vi "StopCore.vi"(8 "error in (no error)":errorcluster caption="错误输入（无错误）", 11 "zsActor输入":refnum<class "ActorWrapper.lvclass">) -> (0 "error out":errorcluster caption="错误输出", 3 "zsActor输出":refnum<class "ActorWrapper.lvclass">)   [LabVIEW 2014]
uses:
  zsActor/ActorWrapper.lvclass
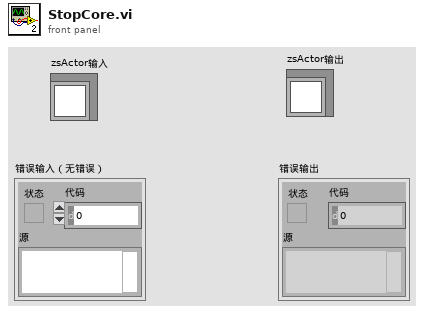
[diagram p1: front panel]
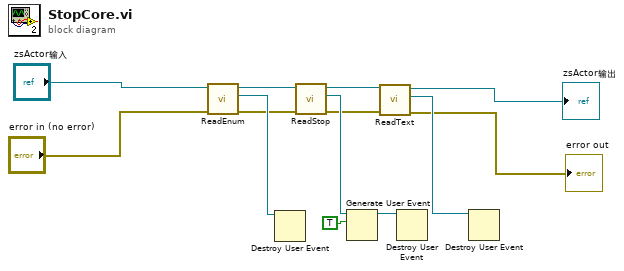
[diagram p0: block diagram]
diagram:
  n1 = call-dynamic "ReadEnum.vi"("error in (no error)"="error in (no error)", "zsActor输入"="zsActor输入") -> ("error out"=w3:errorcluster, "Enum"=w9:refnum<user-event>, "zsActor输出"=w13:refnum<class "ActorWrapper.lvclass">)  [unwired: 7 in]
  n2 = Destroy User Event(user event=w9) -> ()  [unwired: 1 in, 1 out]
  n3 = call-dynamic "ReadStop.vi"("error in (no error)"=w3, "zsActor输入"=w13) -> ("error out"=w2:errorcluster, "Stop"=w8:refnum<user-event>, "zsActor输出"=w12:refnum<class "ActorWrapper.lvclass">)  [unwired: 7 in]
  n4 = Generate User Event(user event=w8, event data cluster=TRUE ("event data")) -> (user event out=w10:refnum<user-event>)  [unwired: 2 in, 1 out]
  n5 = call-dynamic "ReadText.vi"("error in (no error)"=w2, "zsActor输入"=w12) -> ("error out"=→"error out":errorcluster, "Text"=w7:refnum<user-event>, "zsActor输出"=→"zsActor输出":refnum<class "ActorWrapper.lvclass">)  [unwired: 7 in]
  n6 = Destroy User Event(user event=w10) -> ()  [unwired: 1 in, 1 out]
  n7 = Destroy User Event(user event=w7) -> ()  [unwired: 1 in, 1 out]
